vi "Revision Query.vi"(0 "VISA resource name":refnum<visa-resource-name>, 11 "error in (no error)":errorcluster) -> (4 "VISA resource name out":refnum<visa-resource-name>, 6 "Instrument Serial Number":string, 8 "Instrument Driver Revision":string, 10 "Instrument Firmware Revision":string, 14 "Instrument Model Number":string, 15 "error out":errorcluster)   [LabVIEW 2018, in "Lake Shore 372.lvlib"]
doc: "Queries the current instrument firmware revision and instrument driver revision.\n\nRefer to the Readme file for detailed driver information including modification history."
uses:
  Lake Shore 372.lvlib
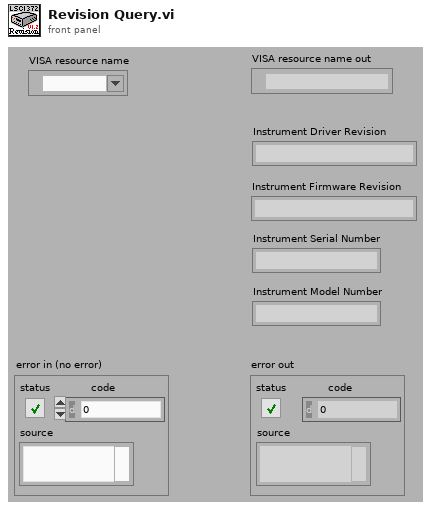
[diagram p1: front panel]
types:
  T1 = cluster{"Major":u16, "Minor":u16, "Fix":u16, "Build":u16}
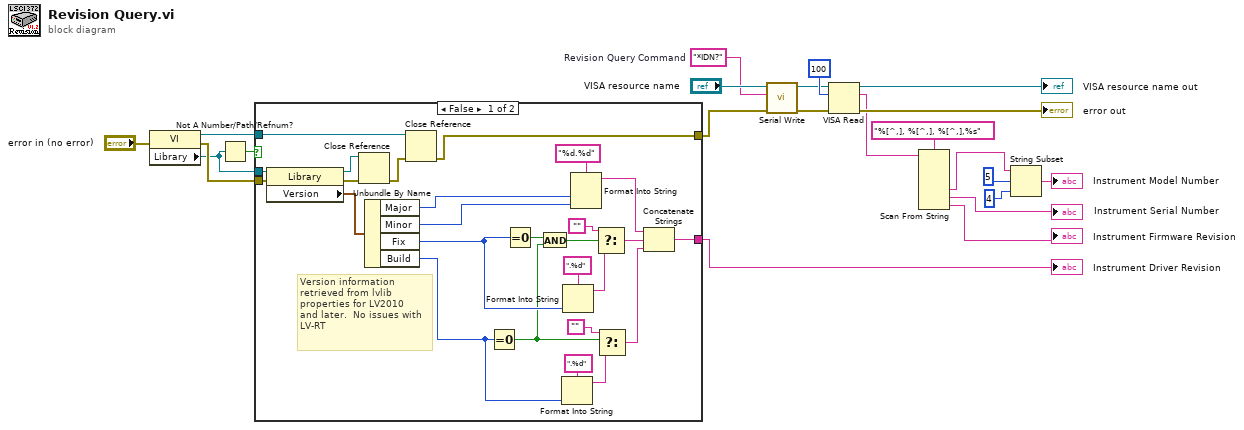
[diagram p0: block diagram]
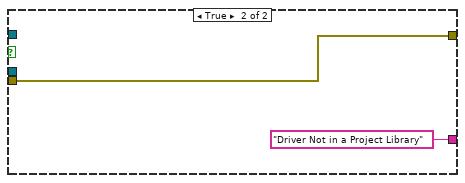
[diagram p2: hidden frame]
diagram:
  w16 = "*IDN?"  # Revision Query Command
  n1 = property class="VI"(error in="error in (no error)") -> (reference out=w4:refnum<vi>, error out=w3:errorcluster, "Library"=w2:refnum<vi>)  [unwired: 1 in]
  n2 = Not A Number/Path/Refnum?(number/path/refnum=w2) -> (NaN/Path/Refnum?=w1:bool)
  n3 = case shown="False" w1 {
    tunnel: w4 -> [w45 _]
    tunnel: w3 -> [w32 w50]
    tunnel: [w28 w50] -> w5
    tunnel: [w27 "Driver Not in a Project Library"] -> w7
    tunnel: w2 -> [w26 _]
    frame False {
      # "Version information\nretrieved from lvlib\nproperties for LV2010\nand later.  No issues with\nLV-RT"
      n4 = property class="Library"(reference=w26, error in=w32) -> (reference out=w47:refnum<vi>, error out=w48:errorcluster, "Version"=w44:T1)
      n5 = Close Reference(reference=w47, error in (no error)=w48) -> (error out=w46:errorcluster)
      n6 = Unbundle By Name(w44) -> ("Major"=w35:u16, "Minor"=w34:u16, "Fix"=w31:u16, "Build"=w33:u16)
      n7 = Close Reference(reference=w45, error in (no error)=w46) -> (error out=w28:errorcluster)
      n8 = Equal To 0?(x=w33) -> (x = 0?=w24:bool)
      n9 = Equal To 0?(x=w31) -> (x = 0?=w30:bool)
      n10 = And(x=w30, y=w24) -> (x .and. y?=w29:bool)
      n11 = Format Into String(format string=".%d", w33) -> (resulting string=w38:string)  [unwired: 2 in, 1 out]
      n12 = Format Into String(format string=".%d", w31) -> (resulting string=w42:string)  [unwired: 2 in, 1 out]
      n13 = Format Into String(format string="%d.%d", w35, w34) -> (resulting string=w40:string)  [unwired: 2 in, 1 out]
      n14 = Select(t="", s=w29, f=w42) -> (s? t:f=w39:string)
      n15 = Select(t="", s=w24, f=w38) -> (s? t:f=w36:string)
      n16 = Concatenate Strings(w40, w39, w36) -> (w27:string)
    }
    frame True {
    }
  }
  "Instrument Driver Revision" <- w7
  n17 = call "Serial Write.vi"("error in (no error)"=w5, "Write Buffer (\"\")"=w16, "VISA resource name"="VISA resource name") -> ("error out"=w17:errorcluster, "VISA resource name out"=w18:refnum<visa-resource-name>)  [unwired: 6 in, 1 out]
  n18 = VISA Read(VISA resource name=w18, byte count=u32 100 ("Num Bytes to Read"), error in (no error)=w17) -> (VISA resource name out=→"VISA resource name out":refnum<visa-resource-name>, read buffer=w11:string, error out=→"error out":errorcluster)  [unwired: 1 out]
  n19 = Scan From String(format string="%[^,], %[^,], %[^,],%s", input string=w11) -> (output 2=w14:string, output 3=→"Instrument Serial Number":string, output 4=→"Instrument Firmware Revision":string)  [unwired: 7 in, 3 out]
  n20 = String Subset(string=w14, offset (0)=5, length (rest)=4) -> (substring=→"Instrument Model Number":string)
